vi "U3 eDAC Example.vi"() -> (0 "error out":errorcluster)   [LabVIEW 2021]
panel:
  in  "Binary":bool
  in  "Channel":i32
  in  "FirstFound":bool=TRUE
  in  "Address":string="1"
  out "Error Message":string
  in  "Voltage":dbl format="%.3f"
  # "Updates 1 analog output using the UD easy function eDAC."
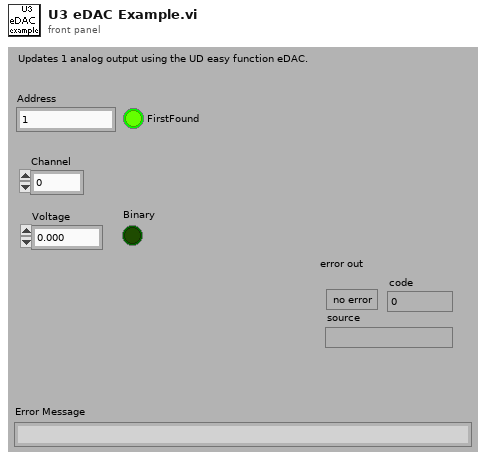
[diagram p1: front panel]
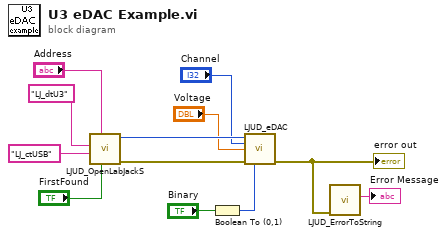
[diagram p0: block diagram]
diagram:
  n1 = call "LJUD_OpenLabJackS.vi"("FirstFound"="FirstFound", "Address"="Address", "ConnectionType"="LJ_ctUSB", "DeviceType"="LJ_dtU3") -> ("error out"=w6:errorcluster, "Handle"=w7:i32)  [unwired: 5 in, 1 out]
  n2 = Boolean To (0,1)(Boolean="Binary") -> (0, 1=w1:i16)
  n3 = call "LJUD_eDAC.vi"("Handle In"=w7, "Channel"="Channel", "Voltage"="Voltage", "error in"=w6, "Binary"=w1) -> ("error out"=w5:errorcluster)  [unwired: 9 in, 1 out]
  "error out" <- w5
  n4 = call "LJUD_ErrorToString.vi"("error in"=w5) -> ("String"=→"Error Message":string)  [unwired: 10 in]
